vi "Spike Function.vi"(1 "x":dbl format="%0.2f") -> (0 "spike(x)":dbl format="%0.2f")   [LabVIEW 2009]
doc: "Generates the spike function for any real number <B>x</B>."
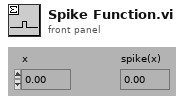
[diagram p1: front panel]
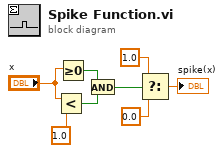
[diagram p0: block diagram]
diagram:
  n1 = Less?(x="x", y=1.0) -> (x < y?=w2:bool)
  n2 = Greater Or Equal To 0?(x="x") -> (x >= 0?=w3:bool)
  n3 = And(x=w3, y=w2) -> (x .and. y?=w1:bool)
  n4 = Select(t=1.0, s=w1, f=0.0) -> (s? t:f=→"spike(x)":dbl)
